vi "READ LASER POWER ORNL Ver1.vi"() -> ()   [LabVIEW 2016]
uses:
  <vilib>/Platform/TimedLoop/XDataNode/timing_clust.ctl
  <vilib>/Platform/TimedLoop/XDataNode/nitl_modes.ctl
  <vilib>/Platform/TimedLoop/XDataNode/wakeup.ctl
  <vilib>/DAQmx/read.llb/DAQmx Read (Digital Bool 1Line 1Point).vi
  <vilib>/DAQmx/read.llb/DAQmx Read (Analog 1D DBL NChan 1Samp).vi
  <vilib>/DAQmx/miscellaneous.llb/DAQmx Fill In Error Info.vi
  <vilib>/platform/TimedLoop/XDataNode/XDataNode.xnode
  <vilib>/Platform/TimedLoop/XDataNode/XDNodeRunTimeDep.lvlib
panel:
  in  "stop":bool
  out "Laser Power kW":dbl
  out "Deposition Trigger":bool
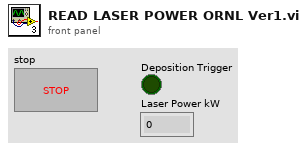
[diagram p1: front panel]
types:
  T1 = typedef "XDNodeRunTimeDep.lvlib/timing_clust.ctl" = cluster{"Expected End [f-1]":u64, "Actual End [f-1]":u64, "Finished Late? [f-1]":bool, "Expected End [i-1]":u64, "Actual End [i-1]":u64, "Finished Late? [i-1]":bool, "Expected Start [i]":u64, "Actual Start [i]":u64, "Expected Start [f]":u64, "Actual Start [f]":u64, "Source Name":string, "Structure Name":string, "Period":i64, "Deadline":i64, "Offset":i64, "Start":i64, "Priority":i32, "Timeout":i32, "Mode":T2, "Wakeup Reason":T3, "Error":errorcluster, "Source Type":string, "Secondary Source Type":string, "Global End Time":u64, "Global Start Time":u64, "Frame Duration":u64, "Iteration Duration":u64, "Assigned CPU":i32, "I/O Scan Engine Mode":u32}
  T2 = typedef "XDNodeRunTimeDep.lvlib/nitl_modes.ctl" = enum32{"No Change", "Process missed periods, maintain original phase", "Discard missed periods, maintain original phase", "Process missed periods, ignore original phase", "Discard missed periods, ignore original phase"}
  T3 = typedef "XDNodeRunTimeDep.lvlib/wakeup.ctl" = enum32{"Normal", "Aborted", "Asynchronous wakeup", "Timing source error", "Timed loop error", "Timeout"}
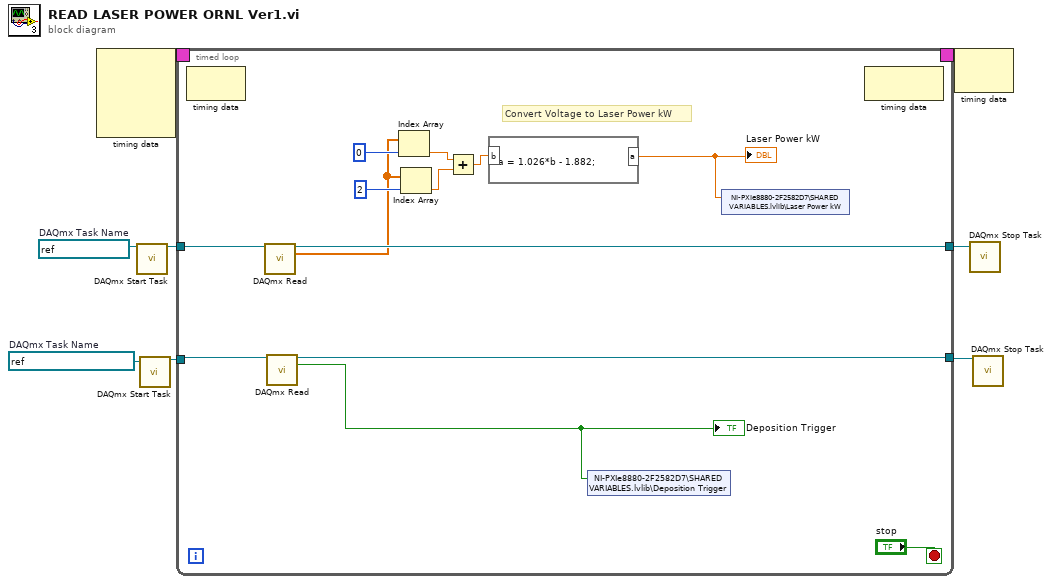
[diagram p0: block diagram]
diagram:
  w3 = refnum<k21> "Deposition Trigger"  # DAQmx Task Name
  w6 = refnum<k21> "Laser Power"  # DAQmx Task Name
  n1 = node-c288() -> (w8:T1)  [unwired: 4 in]
  n2 = call <vilib>:"DAQmx Start Task.vi"("task/channels in"=w6) -> ("task out"=w5:refnum<k21>)  [unwired: 13 in, 1 out]
  n3 = call <vilib>:"DAQmx Start Task.vi"("task/channels in"=w3) -> ("task out"=w2:refnum<k21>)  [unwired: 13 in, 1 out]
  n4 = timed-loop {
    timing: w8 -> [_]
    timing-out: [_] -> w7
    tunnel: w5 -> [w21]
    tunnel: [w20] -> w4
    tunnel: w2 -> [w19]
    tunnel: [w18] -> w1
    stop <- "stop" stop-if-true
    # "Convert Voltage to Laser Power kW"
    n5 = node-c288() -> ()  [unwired: 1 in, 1 out]
    n6 = call-poly <vilib>:"DAQmx Read.vi"("task/channels in"=w21) -> ("task out"=w20:refnum<k21>, "data"=w9:dbl[])  [unwired: 12 in, 1 out]
    n7 = call-poly <vilib>:"DAQmx Read.vi"("task/channels in"=w19) -> ("task out"=w18:refnum<k21>, "data"=w16:bool)  [unwired: 12 in, 1 out]
    "Deposition Trigger" <- w16
    n8 = Index Array(array=w9, index=0) -> (element=w12:dbl)
    n9 = Index Array(array=w9, index=2) -> (element=w11:dbl)
    n10 = Add(x=w12, y=w11) -> (x+y=w10:dbl)
    n11 = formula code="a = 1.026*b - 1.882;"("b"=w10) -> ("a"=w17:dbl)
    "Laser Power kW" <- w17
    n12 = shared-variable "NI-PXIe8880-2F2582D7\\SHARED VARIABLES.lvlib\\Deposition Trigger"(w16) -> ()  [unwired: 1 in, 1 out]
    n13 = shared-variable "NI-PXIe8880-2F2582D7\\SHARED VARIABLES.lvlib\\Laser Power kW"(w17) -> ()  [unwired: 1 in, 1 out]
    n14 = node-c288() -> ()  [unwired: 1 in, 1 out]
  }
  n15 = node-c288(w7) -> ()  [unwired: 1 out]
  n16 = call <vilib>:"DAQmx Stop Task.vi"("task/channels in"=w4) -> ()  [unwired: 13 in, 2 out]
  n17 = call <vilib>:"DAQmx Stop Task.vi"("task/channels in"=w1) -> ()  [unwired: 13 in, 2 out]
